vi "Circle Buffer.vi"   [LabVIEW 2017]
doc: "Polymorphic wrapper that collects incoming samples into a circular buffer of #Count elements. Select the instance for a single sample per call or the one for an array of samples."
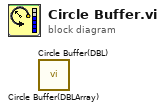
[diagram p0: block diagram]
diagram:
  n1 = call "Circle Buffer(DBLArray).vi"() -> ()  [unwired: 9 in, 1 out]
  n2 = call "Circle Buffer(DBL).vi"() -> ()  [unwired: 8 in, 2 out]
